vi "Main.vi"(11 "Module Admin":refnum<class "Delacor_lib_QMH_Module Admin.lvclass">) -> ()   [LabVIEW 2020, in "TCP Server.lvlib"]
doc: "This template is based off of the Queued Message Handler design pattern and the Queued Message Handler project template that ships with LabVIEW.\n\nThe main difference is that the queue is private to this module and communication between modules is performed via Broadcast and Request events.\n\nRequest events are wrapped in public API methods and are handled in the Event Handling Loop (EHL) of this VI. Any module can register for Broadcast events sent by this module. The EHL generates messages based on user interface actions.\n\nThe Message Handling Loop (MHL) processes messages generated by the EHL, or by other messages. The messages are string values, so new messages can be added easily to the Message Cases case structure in the MHL. Each message cluster can also provide an optional value for Message Data, which is a variant that can be converted to whatever message-specific data is required.\n_____\nBased on DQMH Project Template 6.0.0.91."
uses:
  TCP Server.lvlib
  <vilib>/Delacor/Delacor QMH/Libraries/Module Admin_class/Delacor_lib_QMH_Module Admin.lvclass
  Module Data--cluster.ctl
  <vilib>/Delacor/Delacor QMH/Libraries/Message Queue_class/Delacor_lib_QMH_Message Queue.lvclass/Delacor_lib_QMH_Message Queue.ctl
  Stop Argument--cluster.ctl
  <vilib>/Delacor/Delacor QMH/Libraries/Module Admin_class/Delacor_lib_QMH_Module Admin.lvclass/Delacor_lib_QMH_Module Admin.ctl
  Wake Up Helper Loop Argument--cluster.ctl
  <vilib>/Utility/miscctls.llb/LVPointTypeDef.ctl
  <vilib>/Delacor/Delacor QMH/Libraries/Message Queue_class/Delacor_lib_QMH_Enqueue Message (Single).vi
  <vilib>/Delacor/Delacor QMH/Libraries/Module Admin_class/Delacor_lib_QMH_Get External Launch.vi
  <vilib>/Utility/error.llb/Error Cluster From Error Code.vi
  <vilib>/ErrorRing/Error Ring.xnode
  <vilib>/Delacor/Delacor QMH/Libraries/Message Queue_class/Delacor_lib_QMH_Message Queue.lvclass
panel:
  out "# of Connections":i32
  out "error out":errorcluster
  out "Status":string
  in  "Simulate MHL Error":bool
  in  "Simulate EHL Error":bool
  # "Other QMH Modules communicate with this Module via its Public API (wrappers for its Request Events).\n\nThis Module communicates with other Modules via its Broadcast Events.\nAny module that wants to get these messages, just registers for this module's Broadcast events."
  # "This template is for the Delacor Modified Queued Message Handler design pattern.\n\nSee the block diagram for more information on how to use this template."
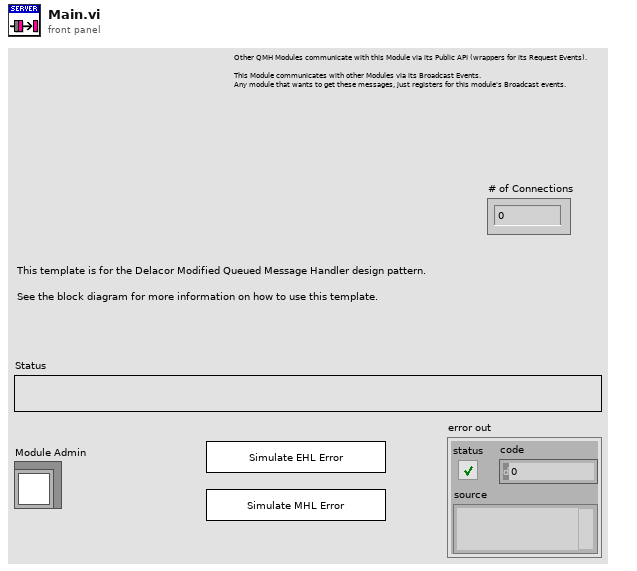
[diagram p1: front panel]
types:
  T1 = typedef "TCP Server.lvlib/Request Events--cluster.ctl" = cluster{"Stop Module":refnum<user-event>, "Show Panel":refnum<user-event>, "Hide Panel":refnum<user-event>, "Get Module Execution Status":refnum<user-event>, "Show Diagram":refnum<user-event>, "Wake Up Helper Loop":refnum<user-event>}
  T2 = typedef "TCP Server.lvlib/Module Data--cluster.ctl" = cluster{"Status":string, "listener ID":refnum<k5>}
  T3 = enum32{"invalid lock state", "Not Locked", "Locked (No Password)", "Password-protected"}
  T4 = typedef "TCP Server.lvlib/Stop Argument--cluster.ctl" = cluster{"Origin":string, "Exit via Stop Module Req?":bool, "Wait for Module to stop?":bool}
  T5 = typedef "TCP Server.lvlib/Wake Up Helper Loop Argument--cluster.ctl" = cluster{"listener":refnum<k5>}
  T6 = typedef "LVPointTypeDef.ctl" = cluster{"Horizontal":i16, "Vertical":i16}
  T7 = enum32{"Invalid", "Standard", "Closed", "Hidden", "Minimized", "Maximized"}
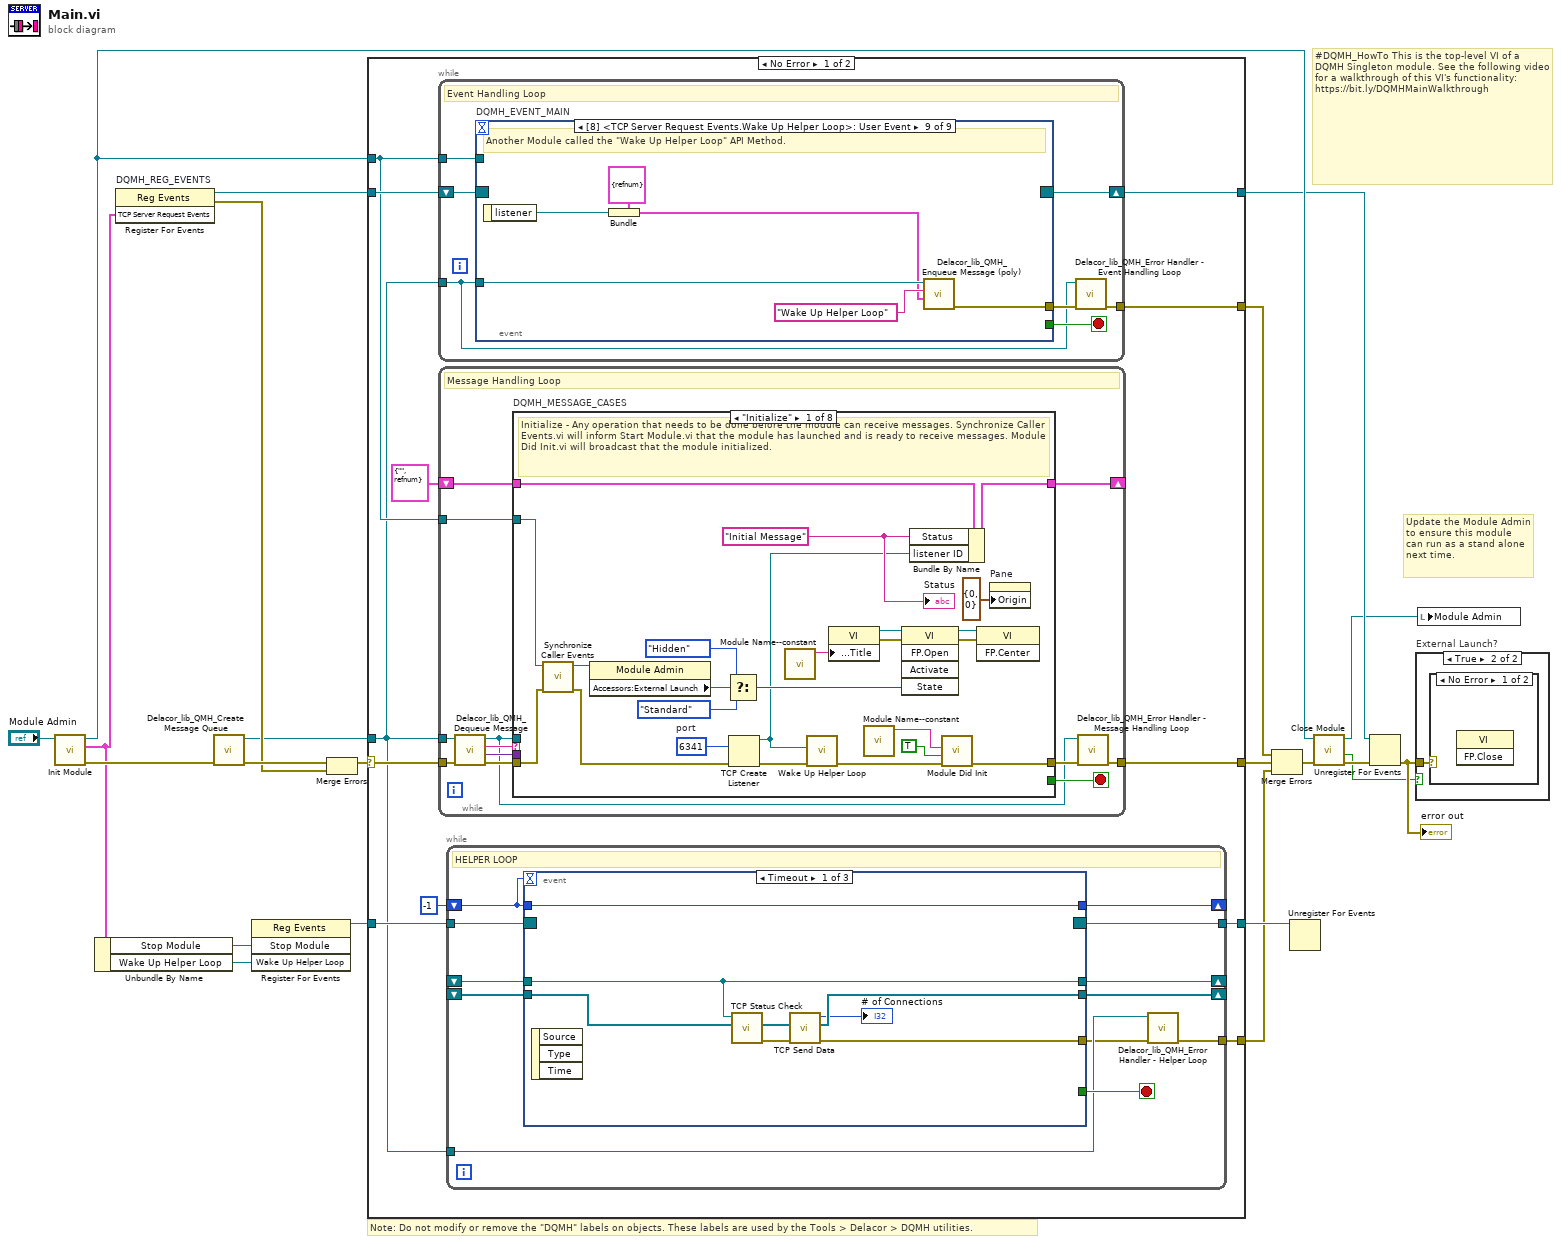
[diagram p0: block diagram]
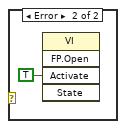
[diagram p3: hidden frame]
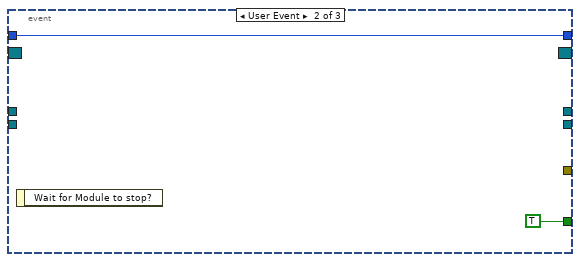
[diagram p4: hidden frame]
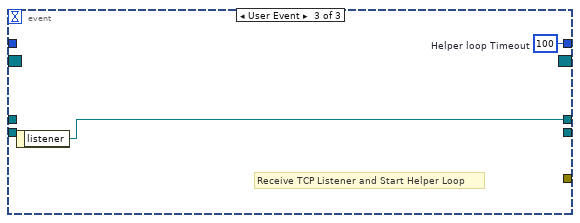
[diagram p5: hidden frame]
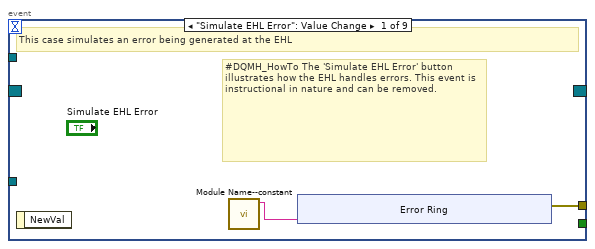
[diagram p6: hidden frame]
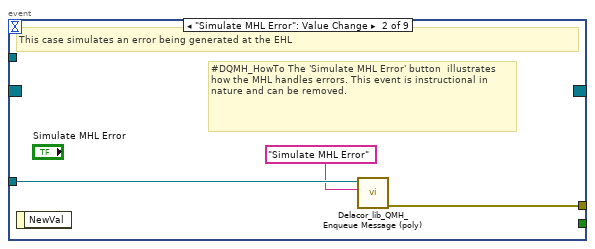
[diagram p7: hidden frame]
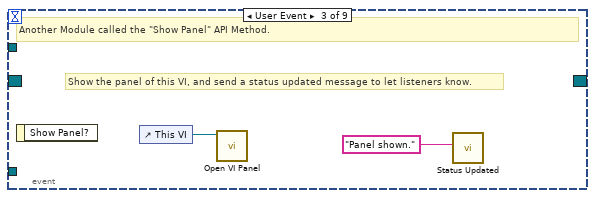
[diagram p8: hidden frame]
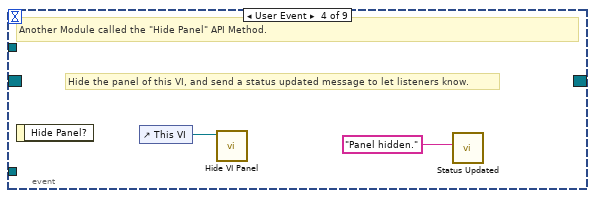
[diagram p9: hidden frame]
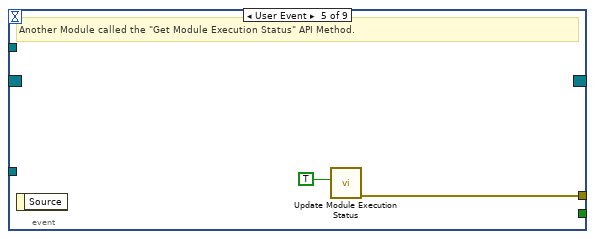
[diagram p10: hidden frame]
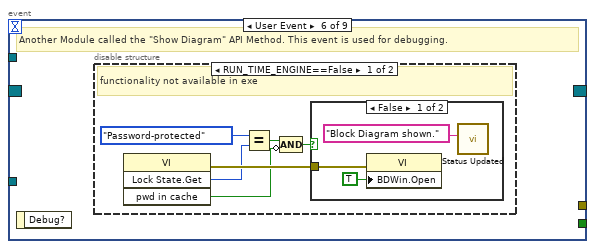
[diagram p11: hidden frame]
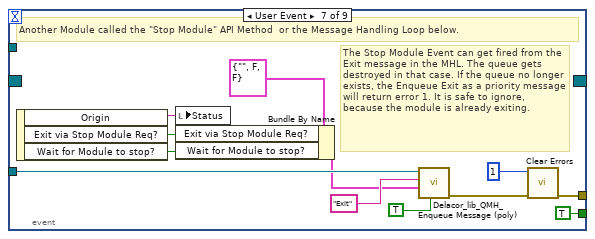
[diagram p14: hidden frame]
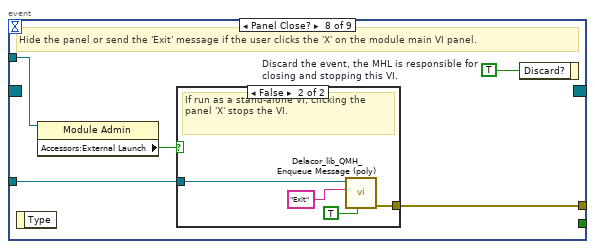
[diagram p15: hidden frame]
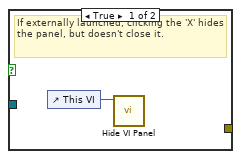
[diagram p16: hidden frame]
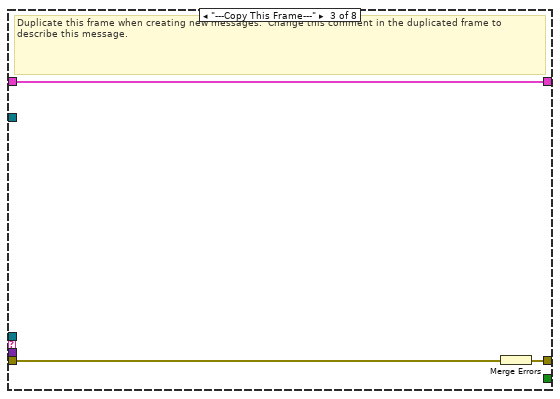
[diagram p18: hidden frame]
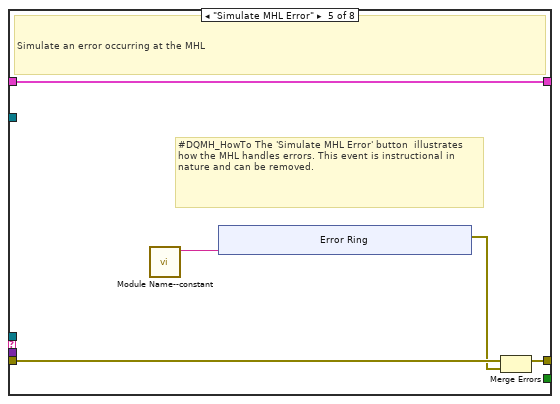
[diagram p20: hidden frame]
diagram:
  # "#DQMH_HowTo This is the top-level VI of a DQMH Singleton module. See the following video for a walkthrough of this VI's functionality: https://bit.ly/DQMHMainWalkthrough"
  # "Note: Do not modify or remove the \"DQMH\" labels on objects. These labels are used by the Tools > Delacor > DQMH utilities."
  # "Update the Module Admin to ensure this module can run as a stand alone next time."
  n1 = call "Init Module.vi"("Singleton Module Admin in"="Module Admin") -> ("error out"=w21:errorcluster, "TCP Server Request Events"=w4:T1, "Singleton Module Admin out"=w13:refnum<class "Delacor_lib_QMH_Module Admin.lvclass">)  [unwired: 8 in]
  n2 = Unbundle By Name(w4) -> ("Stop Module"=w5:refnum<user-event>, "Wake Up Helper Loop"=w1:refnum<user-event>)
  n3 = register-events "DQMH_REG_EVENTS"(w4) -> (reference out=w11:refnum<event-registration>, error out=w14:errorcluster)  [unwired: 2 in]
  n4 = call <vilib>:"Delacor_lib_QMH_Create Message Queue.vi"("error in"=w21) -> ("error out"=w16:errorcluster, "Message Queue"=w10:refnum<class "Delacor_lib_QMH_Message Queue.lvclass">)  [unwired: 9 in]
  n5 = register-events(w5, w1) -> (reference out=w6:refnum<event-registration>)  [unwired: 2 in, 1 out]
  n6 = Merge Errors(w16, w14) -> (w15:errorcluster)
  n7 = case shown="No Error" w15 {
    selector: w15 -> [w32 w224]
    tunnel: [w34 w221] -> w22
    tunnel: [w31 w229] -> w12
    tunnel: w11 -> [w29 w229]
    tunnel: w10 -> [w25 w223]
    tunnel: [w33 _] -> w19
    tunnel: w13 -> [w28 w225]
    tunnel: w6 -> [w27 w222]
    tunnel: [w26 w222] -> w3
    tunnel: [w24 w221] -> w2
    frame No Error {
      n8 = while {
        tunnel: w25 -> [w59]
        shift-right: [w62] -> w31
        shift-left: w29 -> [w63]
        tunnel: [w64] -> w33
        tunnel: w28 -> [w60]
        stop <- w61 stop-if-true
        # "Event Handling Loop"
        n9 = event "DQMH_EVENT_MAIN" shown="[8] <TCP Server Request Events.Wake Up Helper Loop>: User Event" {
          selector: w63 -> [_ _ _ _ _ _ _ _ _]
          dyn-events: [_ _ _ _ _ _ _ _ _] -> w62
          timeout: _ -> [_ _ _ _ _ _ _ _ _]
          tunnel: [_ _ _ _ _ _ TRUE ("Discard?") _ _] -> w61
          tunnel: w59 -> [_ w76 _ _ _ _ w100 w107 w120]
          tunnel: [w67 w77 _ _ w83 _ w103 w109 w115] -> w65
          tunnel: w60 -> [_ _ _ _ _ _ _ w106 _]
          event "Simulate EHL Error": Value Change {
            # "#DQMH_HowTo The 'Simulate EHL Error' button  illustrates how the EHL handles errors. This event is instructional in nature and can be removed."
            # "This case simulates an error being generated at the EHL"
            n10 = event-data() -> ()  [unwired: 1 in, 1 out]
            n11 = call "Module Name--constant.vi"() -> ("Module Name"=w66:string)  [unwired: 11 in]
            n12 = xnode "Error Ring"("parameter 0"=w66) -> ("error out"=w67:errorcluster)
          }
          event "Simulate MHL Error": Value Change {
            # "#DQMH_HowTo The 'Simulate MHL Error' button  illustrates how the MHL handles errors. This event is instructional in nature and can be removed."
            # "This case simulates an error being generated at the EHL"
            n13 = event-data() -> ()  [unwired: 1 in, 1 out]
            n14 = call-poly <vilib>:"Delacor_lib_QMH_Enqueue Message (poly).vi"("Message"="Simulate MHL Error", "Message Queue in"=w76) -> ("error out"=w77:errorcluster)  [unwired: 8 in, 1 out]
          }
          event User Event {
            # "Show the panel of this VI, and send a status updated message to let listeners know."
            # "Another Module called the \"Show Panel\" API Method."
            n15 = event-data() -> ()  [unwired: 1 in, 1 out]
            n16 = control-ref of="This VI"() -> (w79:refnum<vi>)
            n17 = call "Open VI Panel.vi"("VI"=w79) -> ()  [unwired: 10 in, 1 out]
            n18 = call "Status Updated.vi"("Status"="Panel shown." ("format string")) -> ()  [unwired: 10 in, 1 out]
          }
          event User Event {
            # "Hide the panel of this VI, and send a status updated message to let listeners know."
            # "Another Module called the \"Hide Panel\" API Method."
            n19 = event-data() -> ()  [unwired: 1 in, 1 out]
            n20 = control-ref of="This VI"() -> (w81:refnum<vi>)
            n21 = call "Hide VI Panel.vi"("VI"=w81) -> ()  [unwired: 10 in, 1 out]
            n22 = call "Status Updated.vi"("Status"="Panel hidden." ("format string")) -> ()  [unwired: 10 in, 1 out]
          }
          event User Event {
            # "Another Module called the \"Get Module Execution Status\" API Method."
            n23 = event-data() -> ()  [unwired: 1 in, 1 out]
            n24 = call "Update Module Execution Status.vi"("Running?"=TRUE) -> ("error out"=w83:errorcluster)  [unwired: 10 in]
          }
          event User Event {
            # "Another Module called the \"Show Diagram\" API Method. This event is used for debugging."
            n25 = event-data() -> ()  [unwired: 1 in, 1 out]
            n26 = disable-structure shown="RUN_TIME_ENGINE==False" {
              frame condition #0 (active) {
                # "functionality not available in exe"
                n27 = invoke class="VI" method="Lock State.Get"() -> (error out=w89:errorcluster, "Get Lock State"=w88:T3, "pwd in cache"=w85:bool)  [unwired: 4 in, 1 out]
                n28 = Equal?(x=T3."Password-protected", y=w88) -> (x = y?=w86:bool)
                n29 = Compound Arithmetic op=AND(w86, invert w85) -> (w84:bool)
                n30 = case shown="False" w84 {
                  tunnel: w89 -> [w92 _]
                  frame False {
                    n31 = property class="VI"(error in=w92, "BDWin.Open"=TRUE ("Block Diagram Window:Open")) -> ()  [unwired: 1 in, 2 out]
                    n32 = call "Status Updated.vi"("Status"="Block Diagram shown." ("format string")) -> ()  [unwired: 10 in, 1 out]
                  }
                  frame True {
                    # "Password-protected VI, and the password is not in the cache. Do not show the diagram."
                  }
                }
              }
              frame condition #1 {
              }
            }
          }
          event User Event {
            # "The Stop Module Event can get fired from the Exit message in the MHL. The queue gets destroyed in that case. If the queue no longer exists, the Enqueue Exit as a priority message will return error 1. It is safe to ignore, because the module is already exiting."
            # "Another Module called the \"Stop Module\" API Method  or the Message Handling Loop below."
            n33 = event-data() -> ("Origin"=w99:string, "Exit via Stop Module Req?"=w95:bool, "Wait for Module to stop?"=w94:bool)  [unwired: 1 in]
            n34 = local write "Status"(w99) -> ()
            n35 = Bundle By Name(cluster=T4 {"Origin"="", "Exit via Stop Module Req?"=FALSE, "Wait for Module to stop?"=FALSE} ("Stop Argument"), "Exit via Stop Module Req?"=w95, "Wait for Module to stop?"=w94) -> (w93:T4)
            n36 = call-poly <vilib>:"Delacor_lib_QMH_Enqueue Message (poly).vi"("Priority Message? (F)"=TRUE, "Message Data"=w93, "Message"="Exit", "Message Queue in"=w100) -> ("error out"=w104:errorcluster)  [unwired: 6 in, 1 out]
            n37 = call <vilib>:"Clear Errors.vi"("error in (no error)"=w104, "specific error code to clear (0: all)"=1) -> ("error out"=w103:errorcluster)  [unwired: 4 in, 1 out]
          }
          event Panel Close? {
            w108 = TRUE  # Discard the event, the MHL is responsible for closing and stopping this VI.
            # "Hide the panel or send the 'Exit' message if the user clicks the 'X' on the module main VI panel."
            n38 = event-data() -> ()  [unwired: 1 in, 1 out]
            n39 = property class="Module Admin"(reference=w106) -> ("Accessors:External Launch"=w105:bool)  [unwired: 1 in, 2 out]
            n40 = case shown="False" w105 {
              tunnel: w107 -> [_ w113]
              tunnel: [_ w114] -> w109
              frame True {
                # "If externally launched, clicking the 'X' hides the panel, but doesn't close it."
                n41 = control-ref of="This VI"() -> (w110:refnum<vi>)
                n42 = call "Hide VI Panel.vi"("VI"=w110) -> ()  [unwired: 10 in, 1 out]
              }
              frame False {
                # "If run as a stand-alone VI, clicking the panel 'X' stops the VI."
                n43 = call-poly <vilib>:"Delacor_lib_QMH_Enqueue Message (poly).vi"("Priority Message? (F)"=TRUE, "Message"="Exit", "Message Queue in"=w113) -> ("error out"=w114:errorcluster)  [unwired: 7 in, 1 out]
              }
            }
            n44 = event-data("Discard?"=w108) -> ()  [unwired: 1 in, 1 out]
          }
          event User Event {
            # "Another Module called the \"Wake Up Helper Loop\" API Method."
            n45 = event-data() -> ("listener"=w116:refnum<k5>)  [unwired: 1 in]
            n46 = Bundle(cluster=T5 {"listener"=refnum} ("Wake Up Helper Loop Argument"), "listener"=w116) -> (w117:T5)
            n47 = call-poly <vilib>:"Delacor_lib_QMH_Enqueue Message (poly).vi"("Message Data"=w117, "Message"="Wake Up Helper Loop", "Message Queue in"=w120) -> ("error out"=w115:errorcluster)  [unwired: 7 in, 1 out]
          }
        }
        n48 = call-dynamic "Delacor_lib_QMH_Error Handler - Event Handling Loop.vi"("error in"=w65, "Message Queue in"=w59) -> ("dup error in"=w64:errorcluster)  [unwired: 8 in, 1 out]
      }
      n49 = while {
        tunnel: w25 -> [w123]
        shift-right: [w127] -> _
        shift-left: T2 {"Status"="", "listener ID"=refnum} ("Data Cluster") -> [w128]
        tunnel: w32 -> [w131]
        tunnel: [w129] -> w34
        tunnel: w28 -> [w121]
        stop <- w126 stop-if-true
        # "Message Handling Loop"
        n50 = call-dynamic "Delacor_lib_QMH_Dequeue Message.vi"("error in"=w131, "Message Queue in"=w123) -> ("error out"=w130:errorcluster, "Message Data"=w124:variant, "Message"=w125:string, "Message Queue out"=w122:refnum<class "Delacor_lib_QMH_Message Queue.lvclass">)  [unwired: 6 in]
        n51 = case "DQMH_MESSAGE_CASES" shown="\"Initialize\"" w125 {
          selector: w125 -> [_ _ _ _ _ _ _ w208]
          tunnel: w122 -> [_ _ _ _ _ w178 w200 _]
          tunnel: w130 -> [w154 w158 w161 w163 w168 w185 w206 w210]
          tunnel: [w153 w158 w160 w163 w167 w181 w203 w211] -> w132
          tunnel: w128 -> [w144 w157 w159 w162 w165 w180 w199 w209]
          tunnel: [w143 w157 w159 w162 w165 w180 w199 w209] -> w127
          tunnel: [_ _ _ _ _ _ w198 _] -> w126
          tunnel: w124 -> [_ _ _ _ _ w179 w197 _]
          tunnel: w121 -> [w145 _ _ _ _ w177 w192 _]
          frame "Initialize" {
            w137 = u16 6341  # port
            w139 = "Initial Message" ("Initial Message")
            # "Initialize - Any operation that needs to be done before the module can receive messages. Synchronize Caller Events.vi will inform Start Module.vi that the module has launched and is ready to receive messages. Module Did Init.vi will broadcast that the module initialized."
            n52 = call "Synchronize Caller Events.vi"("error in (no error)"=w154, "Singleton Module Admin in"=w145) -> ("error out"=w136:errorcluster, "Singleton Module Admin out"=w140:refnum<class "Delacor_lib_QMH_Module Admin.lvclass">)  [unwired: 8 in]
            n53 = property class="Module Admin"(reference=w140) -> ("Accessors:External Launch"=w149:bool)  [unwired: 1 in, 2 out]
            n54 = Select(t=T7."Hidden" ("State"), s=w149, f=T7."Standard" ("State")) -> (s? t:f=w146:T7)
            n55 = TCP Create Listener(8:w136, 10:w137) -> (0:w135:errorcluster, 3:w133:refnum<k5>)  [unwired: 4 out]
            n56 = call "Module Name--constant.vi"() -> ("Module Name"=w152:string)  [unwired: 11 in]
            n57 = call "Wake Up Helper Loop.vi"("error in"=w135, "listener"=w133) -> ("error out"=w134:errorcluster)  [unwired: 9 in]
            n58 = property class="VI"("Front Panel.Title"=w152) -> (reference out=w151:refnum<vi>, error out=w156:errorcluster)  [unwired: 2 in]
            n59 = call "Module Name--constant.vi"() -> ("Module Name"=w141:string)  [unwired: 11 in]
            n60 = invoke class="VI" method="FP.Open"(reference=w151, error in=w156, "State"=w146) -> (reference out=w150:refnum<vi>, error out=w155:errorcluster)  [unwired: 2 in, 3 out]
            n61 = Bundle By Name(cluster=w144, "Status"=w139, "listener ID"=w133) -> (w143:T2)
            n62 = call "Module Did Init.vi"("error in (no error)"=w134, "Initialized?"=TRUE, "Origin"=w141) -> ("error out"=w153:errorcluster)  [unwired: 8 in]
            n63 = invoke class="VI" method="FP.Center"(reference=w150, error in=w155) -> ()  [unwired: 1 in, 3 out]
            n64 = property on="Pane" class="Pane"("Origin"=T6 {"Horizontal"=0, "Vertical"=0}) -> ()  [unwired: 2 in, 2 out]
            "Status" <- w139
          }
          frame "---Module Specific---" {
            # "Separator -- The following cases handle messages specific to this Module."
          }
          frame "---Copy This Frame---" {
            # "Duplicate this frame when creating new messages.  Change this comment in the duplicated frame to describe this message."
            n65 = Merge Errors(w161) -> (w160:errorcluster)
          }
          frame "---Exit and Error Handling---" {
            # "Separator - The following cases handle errors and exit messages."
          }
          frame "Simulate MHL Error" {
            # "#DQMH_HowTo The 'Simulate MHL Error' button  illustrates how the MHL handles errors. This event is instructional in nature and can be removed."
            # "Simulate an error occurring at the MHL"
            n66 = call "Module Name--constant.vi"() -> ("Module Name"=w164:string)  [unwired: 11 in]
            n67 = xnode "Error Ring"("parameter 0"=w164) -> ("error out"=w166:errorcluster)
            n68 = Merge Errors(w168, w166) -> (w167:errorcluster)
          }
          frame "Error" {
            # "#CodeRecommended - If you ever change the name of this \"Error\" message, you'll need to update the name in the Check Loop Error.vi as well."
            # "#CodeRecommended - If the module is running in standalone mode (External Launch = FALSE), this code will pop up an error dialog and call the 'Exit' message if an error occurs. Add more fine-grained error handling here."
            # "Error - Check the error message data and respond accordingly. This message is sent by the \"Error Handler\" VIs at the end of each loop in this application."
            n69 = property class="Module Admin"(reference=w177) -> ("Accessors:External Launch"=w176:bool)  [unwired: 1 in, 2 out]
            n70 = Variant To Data(error in=w185, type=errorcluster {"status"=FALSE, "code"=0, "source"=""} ("error constant"), Variant=w179) -> (data=w186:errorcluster, error out=w183:errorcluster)
            n71 = call "Error Reported.vi"("Error"=w186) -> ()  [unwired: 10 in, 1 out]
            n72 = case shown="False" w176 {
              tunnel: [w191 _] -> w182
              tunnel: w178 -> [w189 _]
              tunnel: w186 -> [w190 _]
              frame False {
                # "If the module is running standalone, then pop up an error dialog and call the \"Exit\" message."
                n73 = call <vilib>:"Simple Error Handler.vi"("error in (no error)"=w190) -> ()  [unwired: 4 in, 5 out]
                n74 = call-poly <vilib>:"Delacor_lib_QMH_Enqueue Message (poly).vi"("Priority Message? (F)"=TRUE, "Message"="Exit", "Message Queue in"=w189) -> ("error out"=w191:errorcluster)  [unwired: 7 in, 1 out]
              }
              frame True {
                # "If the module was launched externally, calling the Error Reported broadcast VI is the only action performed by the \"Error\" message. The module's caller can then process the error appropriately."
              }
            }
            n75 = Merge Errors(w183, w182) -> (w181:errorcluster)
            n76 = local write "error out"(w181) -> ()
          }
          frame "Exit" {
            w196 = 91  # 91: not all Exit messages will have an argument
            w198 = TRUE  # Stop the VI
            # "Release the message queue reference"
            # "#CodeNeeded - Add any required cleanup code here"
            # "Exit - Exit the application."
            n77 = Variant To Data(error in=w206, type=T4 {"Origin"="", "Exit via Stop Module Req?"=FALSE, "Wait for Module to stop?"=FALSE} ("Stop Argument"), Variant=w197) -> (data=w194:T4, error out=w202:errorcluster)
            n78 = call <vilib>:"Clear Errors.vi"("error in (no error)"=w202, "specific error code to clear (0: all)"=w196) -> ("error out"=w205:errorcluster)  [unwired: 4 in, 1 out]
            n79 = control-ref of="This VI"() -> (w193:refnum<vi>)
            n80 = call-dynamic "Delacor_lib_QMH_Release Message Queue.vi"("error in"=w205, "Message Queue"=w200) -> ("error out"=w204:errorcluster)  [unwired: 9 in]
            n81 = call "Handle Exit.vi"("Stop Argument"=w194, "Admin in"=w192, "VI reference"=w193) -> ("error out"=w201:errorcluster)  [unwired: 7 in, 1 out]
            n82 = Merge Errors(w204, w201) -> (w203:errorcluster)
          }
          frame Default {
            # "'Default' case only runs if there is a message that isn't defined in any of the other cases.  Output a programming error."
            n83 = call "Module Name--constant.vi"() -> ("Module Name"=w207:string)  [unwired: 11 in]
            n84 = xnode "Error Ring"("parameter 0"=w208, "parameter 1"=w207) -> ("error out"=w212:errorcluster)
            n85 = Merge Errors(w210, w212) -> (w211:errorcluster)
          }
        }
        n86 = call-dynamic "Delacor_lib_QMH_Error Handler - Message Handling Loop.vi"("error in"=w132, "Message Queue in"=w122) -> ("dup error in"=w129:errorcluster)  [unwired: 8 in, 1 out]
      }
      n87 = while {
        tunnel: w27 -> [w46]
        tunnel: [w45] -> w26
        tunnel: w25 -> [w43]
        tunnel: [w42] -> w24
        shift-right: [w41] -> _
        shift-left: _ -> [w40]
        shift-right: [w39] -> _
        shift-left: -1 -> [w38]
        shift-right: [w37] -> _
        shift-left: _ -> [w36]
        stop <- w44 stop-if-true
        # "HELPER LOOP"
        n88 = event shown="[0] Timeout" {
          selector: w46 -> [_ _ _]
          dyn-events: [_ _ _] -> w45
          timeout: w38 -> [_ _ _]
          tunnel: [_ TRUE _] -> w44
          tunnel: [w53 _ w58] -> w41
          tunnel: w40 -> [w53 _ _]
          tunnel: [w54 w55 w57] -> w39
          tunnel: w38 -> [w54 w55 _]
          tunnel: [w50 _ _] -> w37
          tunnel: w36 -> [w52 _ _]
          tunnel: [w47 _ _] -> w35
          event Timeout {
            n89 = event-data() -> ()  [unwired: 1 in, 3 out]
            n90 = call "TCP Status Check.vi"("Clients"=w52, "listener"=w53) -> ("no error"=w49:errorcluster, "Clients"=w51:refnum<k5>[])  [unwired: 7 in, 1 out]
            n91 = call "TCP Send Data.vi"("error in"=w49, "Clients"=w51) -> ("error out"=w47:errorcluster, "Clients"=w50:refnum<k5>[], "# of Connections"=→"# of Connections":i32)  [unwired: 6 in, 1 out]
          }
          event User Event {
            n92 = event-data() -> ()  [unwired: 1 in, 1 out]
          }
          event User Event {
            w57 = 100  # Helper loop Timeout
            # "Receive TCP Listener and Start Helper Loop"
            n93 = event-data() -> ("listener"=w58:refnum<k5>)  [unwired: 1 in]
          }
        }
        n94 = call-dynamic "Delacor_lib_QMH_Error Handler - Helper Loop.vi"("error in"=w35, "Message Queue in"=w43) -> ("dup error in"=w42:errorcluster)  [unwired: 8 in, 1 out]
      }
    }
    frame Error {
      # "Synchronize Caller Events.vi will inform Start Module.vi that the module has launched and will let the code calling Start Module.vi register for broadcasts and would permit the caller receive the broadcast that an error occurred at launch time."
      n95 = call-dynamic "Delacor_lib_QMH_Release Message Queue.vi"("error in"=w224, "Message Queue"=w223) -> ("error out"=w221:errorcluster)  [unwired: 9 in]
      n96 = call "Synchronize Caller Events.vi"("Singleton Module Admin in"=w225) -> ("error out"=w230:errorcluster)  [unwired: 9 in, 1 out]
      n97 = call "Module Name--constant.vi"() -> ("Module Name"=w228:string)  [unwired: 11 in]
      n98 = Format Into String(format string="An error occurred during initialization. %s is no longer running.", w228) -> (resulting string=w226:string)  [unwired: 2 in, 1 out]
      n99 = Merge Errors(w221, w230) -> (w231:errorcluster)
      n100 = call "Error Reported.vi"("Additional Information"=w226, "Error"=w231) -> ()  [unwired: 9 in, 1 out]
    }
  }
  n101 = Merge Errors(w19, w22, w2) -> (w18:errorcluster)
  n102 = Unregister For Events(event registration refnum=w3) -> ()  [unwired: 1 in, 1 out]
  n103 = call "Close Module.vi"("error in (no error)"=w18, "Module Admin in"=w13) -> ("error out"=w20:errorcluster, "External Launch"=w7:bool, "Module Admin out"=w8:refnum<class "Delacor_lib_QMH_Module Admin.lvclass">)  [unwired: 7 in]
  n104 = Unregister For Events(event registration refnum=w12, error in=w20) -> (error out=w17:errorcluster)
  "error out" <- w17
  n105 = case "External Launch?" shown="True" w7 {
    tunnel: w17 -> [_ w232]
    frame False {
    }
    frame True {
      n106 = case shown="No Error" w232 {
        frame No Error {
          n107 = invoke class="VI" method="FP.Close"() -> ()  [unwired: 3 in, 3 out]
        }
        frame Error {
          n108 = invoke class="VI" method="FP.Open"("Activate"=TRUE ("Activate?")) -> ()  [unwired: 4 in, 5 out]
        }
      }
    }
  }
  n109 = local write "Module Admin"(w8) -> ()
